vi "Wybor rejestratora.vi"(8 "error in (no error)":errorcluster, 11 "Konfiguracja in":path=path "C:/Users/user/Documents/Rudpol2/Konfiguracja") -> (0 "error out":errorcluster, 2 "Plik":string)   [LabVIEW 2014]
doc: "Wybiera plik konfiguracyjny dla kanałów analogowych\ndla podłączonego rejestratora"
uses:
  <vilib>/Utility/miscctls.llb/LVStringsAndValuesArrayTypeDef_U16.ctl
panel:
  in  "Urzadzenie":u16(ring) caption="Wybierz Urządzenie" items=["REJESTRATOR 1.jnj", "REJESTRATOR 10.jnj", "REJESTRATOR 2.jnj", "REJESTRATOR 3.jnj"]
  in  "OK Button":bool
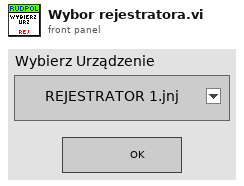
[diagram p1: front panel]
types:
  T1 = typedef "LVStringsAndValuesArrayTypeDef_U16.ctl" = cluster{"String":string, "Value":u16}[]
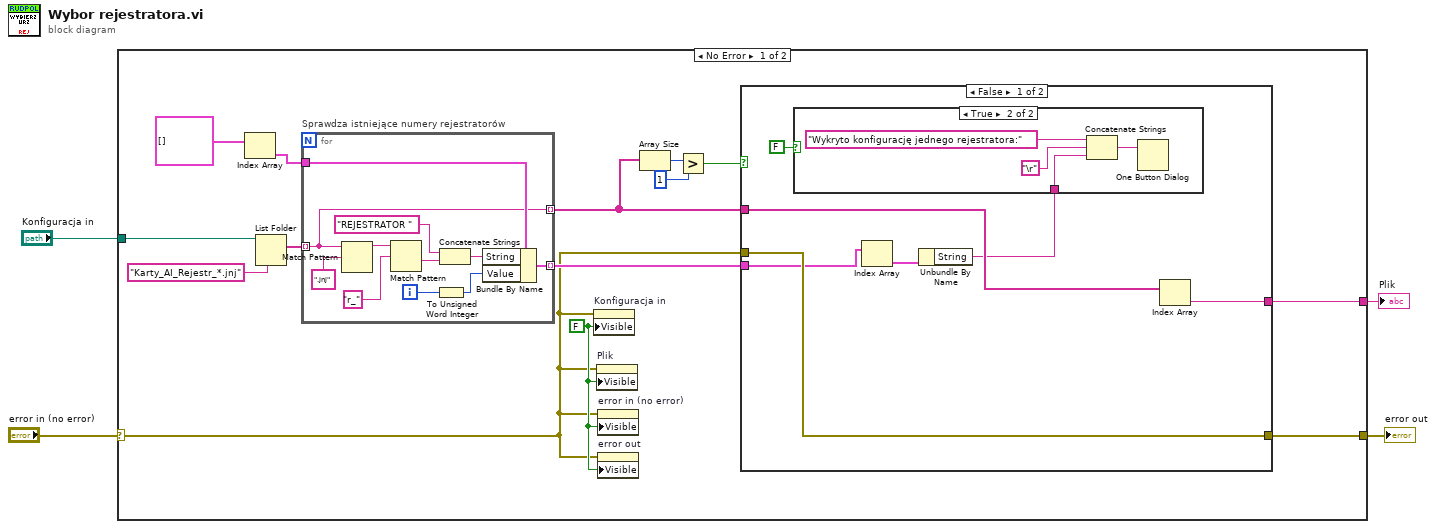
[diagram p0: block diagram]
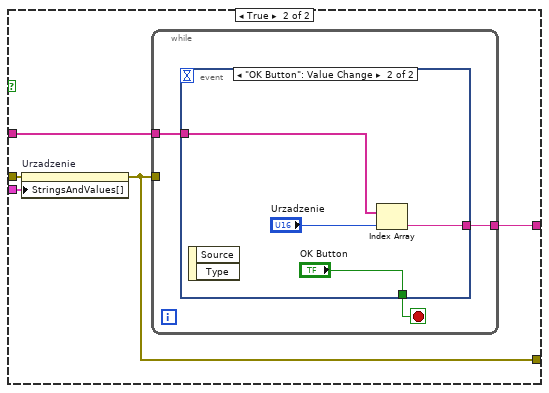
[diagram p3: hidden frame]
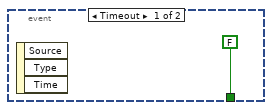
[diagram p4: hidden frame]
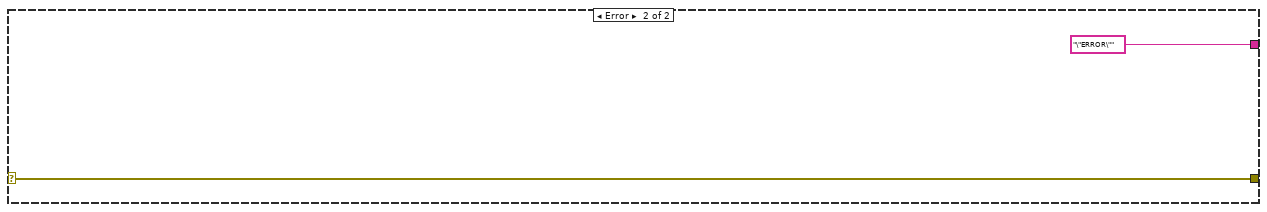
[diagram p5: hidden frame]
diagram:
  n1 = case shown="No Error" "error in (no error)" {
    selector: "error in (no error)" -> [w9 w54]
    tunnel: "Konfiguracja in" -> [w17 _]
    tunnel: [w13 "\"ERROR\""] -> w3
    tunnel: [w11 w54] -> w1
    frame No Error {
      w10 = FALSE ("Visible")
      n2 = Index Array(array=T1 [] ("Strings And Values []")) -> (element=w15:cluster{"String":string, "Value":u16})  [unwired: 1 in]
      n3 = List Folder(path=w17, pattern="Karty_AI_Rejestr_*.jnj") -> (filenames=w12:string[])  [unwired: 2 in, 3 out]
      n4 = for "Sprawdza istniejące numery rejestratorów" {
        tunnel: w12 -> [w43] mode=indexing
        tunnel: [w48] -> w14 mode=indexing
        tunnel: w15 -> [w44]
        tunnel: [w43] -> w8 mode=indexing
        i -> [w47]
        n5 = Match Pattern(string=w43, regular expression=".jnj") -> (before substring=w52:string)  [unwired: 1 in, 3 out]
        n6 = Match Pattern(string=w52, regular expression="r_") -> (after substring=w50:string)  [unwired: 1 in, 3 out]
        n7 = To Unsigned Word Integer(number=w47) -> (unsigned 16bit integer=w46:u16)
        n8 = Concatenate Strings("REJESTRATOR " ("regular expression"), w50) -> (w45:string)
        n9 = Bundle By Name(cluster=w44, "String"=w45, "Value"=w46) -> (w48:cluster{"String":string, "Value":u16})
      }
      n10 = property on="Konfiguracja in" class="Path"(error in=w9, "Visible"=w10) -> ()  [unwired: 1 in, 2 out]
      n11 = property on="Plik" class="Str"(error in=w9, "Visible"=w10) -> ()  [unwired: 1 in, 2 out]
      n12 = property on="error in (no error)" class="Clust (strict)"(error in=w9, "Visible"=w10) -> ()  [unwired: 1 in, 2 out]
      n13 = property on="error out" class="Clust (strict)"(error in=w9, "Visible"=w10) -> ()  [unwired: 1 in, 2 out]
      n14 = Array Size(array=w8) -> (size(s)=w7:i32)
      n15 = Greater?(x=w7, y=1) -> (0:w5:bool)
      n16 = case shown="False" w5 {
        tunnel: w8 -> [w23 w34]
        tunnel: w14 -> [w22 w33]
        tunnel: [w24 w32] -> w13
        tunnel: [w25 w31] -> w11
        tunnel: w9 -> [w25 w30]
        frame False {
          n17 = Index Array(array=w22) -> (element=w21:cluster{"String":string, "Value":u16})  [unwired: 1 in]
          n18 = Unbundle By Name(w21) -> ("String"=w20:string)
          n19 = case shown="True" FALSE {
            tunnel: w20 -> [_ w28]
            frame False {
            }
            frame True {
              n20 = Concatenate Strings("Wykryto konfigurację jednego rejestratora:" ("message"), "\r", w28) -> (w27:string)
              n21 = One Button Dialog(message=w27) -> ()  [unwired: 1 in, 1 out]
            }
          }
          n22 = Index Array(array=w23) -> (element=w24:string)  [unwired: 1 in]
        }
        frame True {
          n23 = property on="Urzadzenie" class="Ring (strict)"(error in=w30, "StringsAndValues[]"=w33) -> (error out=w31:errorcluster)  [unwired: 1 in, 1 out]
          n24 = while {
            tunnel: w34 -> [w36]
            tunnel: w31 -> [_]
            tunnel: [w35] -> w32
            stop <- w37 stop-if-true
            n25 = event shown="[1] \"OK Button\": Value Change" {
              selector: _ -> [_ _]
              dyn-events: _ -> [_ _]
              timeout: _ -> [_ _]
              tunnel: [FALSE ("OK Button") "OK Button"] -> w37
              tunnel: w36 -> [_ w40]
              tunnel: [_ w39] -> w35
              event Timeout {
                n26 = event-data() -> ()  [unwired: 1 in, 3 out]
              }
              event "OK Button": Value Change {
                n27 = event-data() -> ()  [unwired: 1 in, 2 out]
                n28 = Index Array(array=w40, index="Urzadzenie") -> (element=w39:string)
              }
            }
          }
        }
      }
    }
    frame Error {
    }
  }
  "Plik" <- w3
  "error out" <- w1
